vi "chart series set pattern.vi"(8 "error in (no error)":errorcluster, 10 "pattern":T1, 11 "series":u32) -> (0 "error out":errorcluster, 2 "pattern out":T1)   [LabVIEW 2015, in "xlsxwriter.lvlib"]
doc: "void chart_series_set_pattern(lxw_chart_series series, lxw_chart_pattern *pattern);"
uses:
  xlsxwriter.lvlib
  xlsxwriter.dll
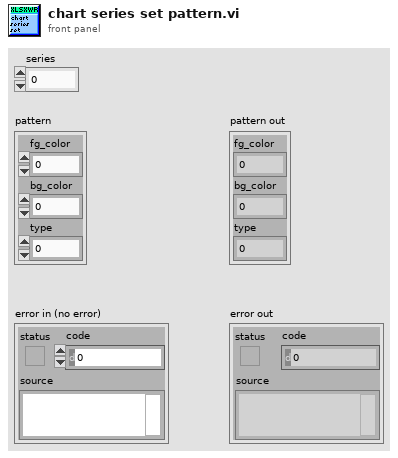
[diagram p1: front panel]
types:
  T1 = cluster{"fg_color":u32, "bg_color":u32, "type":u8}
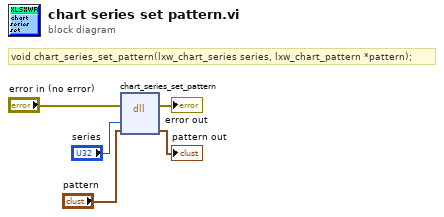
[diagram p0: block diagram]
diagram:
  # "void chart_series_set_pattern(lxw_chart_series series, lxw_chart_pattern *pattern);"
  n1 = dll-call lib="C:/Users/WDAGUtilityAccount/Desktop/lv_vis_added_cell/xlsxwriter.*" fn="chart_series_set_pattern"(error in="error in (no error)", "series"="series", "pattern"="pattern") -> (error out=→"error out":errorcluster, "pattern"=→"pattern out":T1)  [unwired: 4 in, 1 out]
